vi "Condition Init VI.vi"(8 "error in":errorcluster, 9 "Control FP Order":i32[](array[numeric]), 10 "Ref.Init VI":refnum<vi>) -> (0 "error out":errorcluster)   [LabVIEW 2020, in "_Msg Rescript.lvlib" / "_Msg Rescript.lvclass"]
uses:
  _Msg Rescript.lvclass
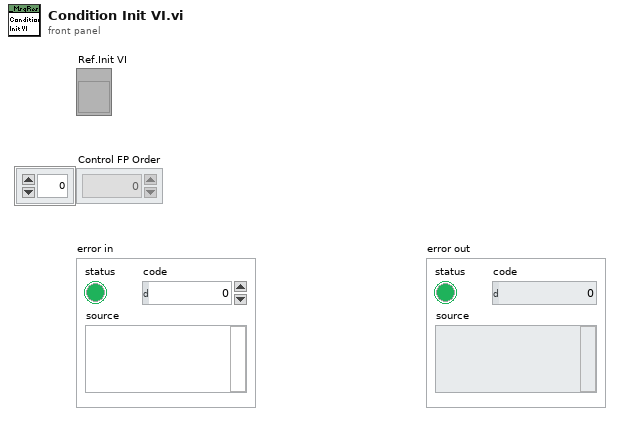
[diagram p1: front panel]
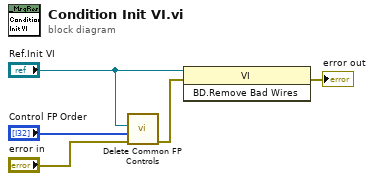
[diagram p0: block diagram]
diagram:
  n1 = call "Delete Common FP Controls.vi"("error in"="error in", "Control FP Order"="Control FP Order", "Ref. VI"="Ref.Init VI") -> ("error out"=w3:errorcluster)  [unwired: 8 in]
  n2 = invoke class="VI" method="BD.Remove Bad Wires"(reference="Ref.Init VI", error in=w3) -> (error out=→"error out":errorcluster)  [unwired: 1 in, 2 out]
